vi "Function_Sort Data Array #.vi"(1 "Data Array In":cluster{"Name":string, "Variant Out":variant}[](array[cluster])) -> (0 "Data Array Out":T1)   [LabVIEW 2013]
uses:
  Control/Control_Data Array.ctl
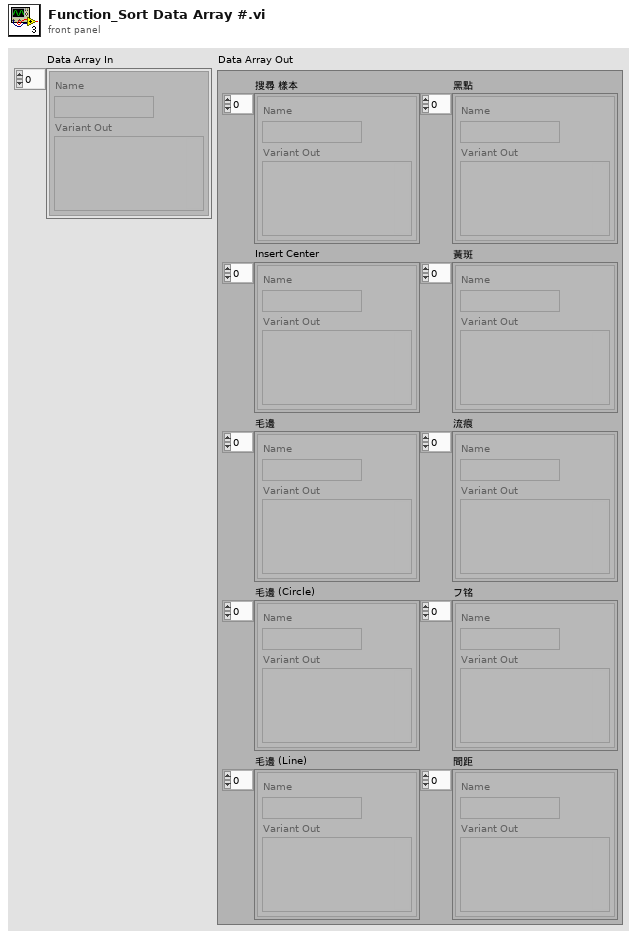
[diagram p1: front panel]
types:
  T1 = typedef "Control_Data Array.ctl" = cluster{"搜尋 樣本":cluster{"Name":string, "Variant Out":variant}[], "Insert Center":cluster{"Name":string, "Variant Out":variant}[], "毛邊":cluster{"Name":string, "Variant Out":variant}[], "毛邊 (Circle)":cluster{"Name":string, "Variant Out":variant}[], "毛邊 (Line)":cluster{"Name":string, "Variant Out":variant}[], "黑點":cluster{"Name":string, "Variant Out":variant}[], "黃斑":cluster{"Name":string, "Variant Out":variant}[], "流痕":cluster{"Name":string, "Variant Out":variant}[], "フ铭":cluster{"Name":string, "Variant Out":variant}[], "間距":cluster{"Name":string, "Variant Out":variant}[]}
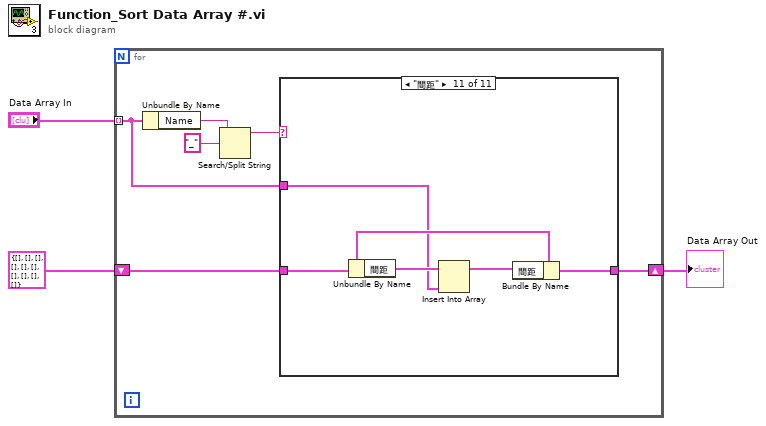
[diagram p0: block diagram]
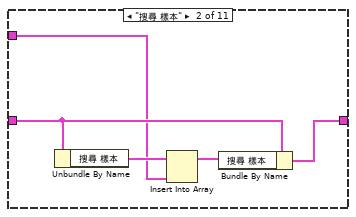
[diagram p3: hidden frame]
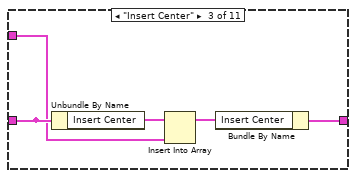
[diagram p4: hidden frame]
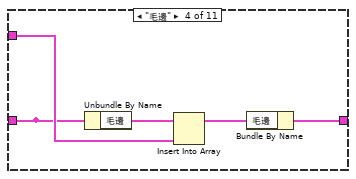
[diagram p5: hidden frame]
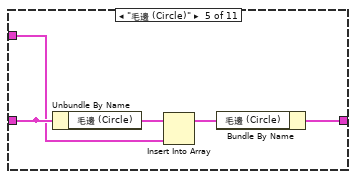
[diagram p6: hidden frame]
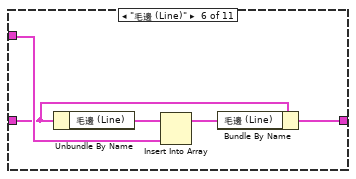
[diagram p7: hidden frame]
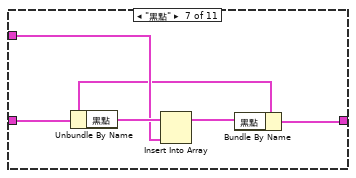
[diagram p8: hidden frame]
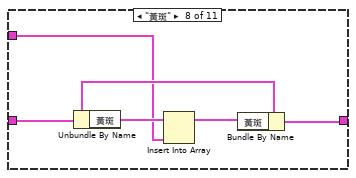
[diagram p9: hidden frame]
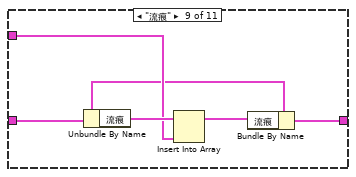
[diagram p10: hidden frame]
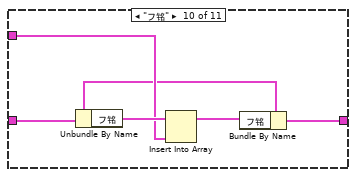
[diagram p11: hidden frame]
diagram:
  n1 = for {
    tunnel: "Data Array In" -> [w7] mode=indexing
    shift-right: [w5] -> w1
    shift-left: T1 {"搜尋 樣本"=[], "Insert Center"=[], "毛邊"=[], "毛邊 (Circle)"=[], "毛邊 (Line)"=[], "黑點"=[], "黃斑"=[], "流痕"=[], "フ铭"=[], "間距"=[]} ("Data Array Out") -> [w6]
    n2 = Unbundle By Name(w7) -> ("Name"=w8:string)
    n3 = Search/Split String(string=w8, search string/char (-)="_") -> (substring before match=w4:string)  [unwired: 1 in, 2 out]
    n4 = case shown="\"間距\"" w4 {
      tunnel: w7 -> [_ w11 w16 w22 w26 w32 w37 w41 w48 w53 w56]
      tunnel: w6 -> [w10 w15 w18 w21 w28 w31 w36 w43 w46 w51 w57]
      tunnel: [w10 w14 w17 w23 w27 w33 w38 w42 w47 w52 w58] -> w5
      frame " - - 選擇檢測項目- - ", Default {
      }
      frame "搜尋 樣本" {
        n5 = Unbundle By Name(w15) -> ("搜尋 樣本"=w13:cluster{"Name":string, "Variant Out":variant}[])
        n6 = Insert Into Array(array=w13, new element=w11) -> (w12:cluster{"Name":string, "Variant Out":variant}[])  [unwired: 1 in]
        n7 = Bundle By Name(cluster=w15, "搜尋 樣本"=w12) -> (w14:T1)
      }
      frame "Insert Center" {
        n8 = Unbundle By Name(w18) -> ("Insert Center"=w20:cluster{"Name":string, "Variant Out":variant}[])
        n9 = Insert Into Array(array=w20, new element=w16) -> (w19:cluster{"Name":string, "Variant Out":variant}[])  [unwired: 1 in]
        n10 = Bundle By Name(cluster=w18, "Insert Center"=w19) -> (w17:T1)
      }
      frame "毛邊" {
        n11 = Unbundle By Name(w21) -> ("毛邊"=w25:cluster{"Name":string, "Variant Out":variant}[])
        n12 = Insert Into Array(array=w25, new element=w22) -> (w24:cluster{"Name":string, "Variant Out":variant}[])  [unwired: 1 in]
        n13 = Bundle By Name(cluster=w21, "毛邊"=w24) -> (w23:T1)
      }
      frame "毛邊 (Circle)" {
        n14 = Unbundle By Name(w28) -> ("毛邊 (Circle)"=w30:cluster{"Name":string, "Variant Out":variant}[])
        n15 = Insert Into Array(array=w30, new element=w26) -> (w29:cluster{"Name":string, "Variant Out":variant}[])  [unwired: 1 in]
        n16 = Bundle By Name(cluster=w28, "毛邊 (Circle)"=w29) -> (w27:T1)
      }
      frame "毛邊 (Line)" {
        n17 = Unbundle By Name(w31) -> ("毛邊 (Line)"=w35:cluster{"Name":string, "Variant Out":variant}[])
        n18 = Insert Into Array(array=w35, new element=w32) -> (w34:cluster{"Name":string, "Variant Out":variant}[])  [unwired: 1 in]
        n19 = Bundle By Name(cluster=w31, "毛邊 (Line)"=w34) -> (w33:T1)
      }
      frame "黑點" {
        n20 = Unbundle By Name(w36) -> ("黑點"=w40:cluster{"Name":string, "Variant Out":variant}[])
        n21 = Insert Into Array(array=w40, new element=w37) -> (w39:cluster{"Name":string, "Variant Out":variant}[])  [unwired: 1 in]
        n22 = Bundle By Name(cluster=w36, "黑點"=w39) -> (w38:T1)
      }
      frame "黃斑" {
        n23 = Unbundle By Name(w43) -> ("黃斑"=w45:cluster{"Name":string, "Variant Out":variant}[])
        n24 = Insert Into Array(array=w45, new element=w41) -> (w44:cluster{"Name":string, "Variant Out":variant}[])  [unwired: 1 in]
        n25 = Bundle By Name(cluster=w43, "黃斑"=w44) -> (w42:T1)
      }
      frame "流痕" {
        n26 = Unbundle By Name(w46) -> ("流痕"=w50:cluster{"Name":string, "Variant Out":variant}[])
        n27 = Insert Into Array(array=w50, new element=w48) -> (w49:cluster{"Name":string, "Variant Out":variant}[])  [unwired: 1 in]
        n28 = Bundle By Name(cluster=w46, "流痕"=w49) -> (w47:T1)
      }
      frame "フ铭" {
        n29 = Unbundle By Name(w51) -> ("フ铭"=w55:cluster{"Name":string, "Variant Out":variant}[])
        n30 = Insert Into Array(array=w55, new element=w53) -> (w54:cluster{"Name":string, "Variant Out":variant}[])  [unwired: 1 in]
        n31 = Bundle By Name(cluster=w51, "フ铭"=w54) -> (w52:T1)
      }
      frame "間距" {
        n32 = Unbundle By Name(w57) -> ("間距"=w60:cluster{"Name":string, "Variant Out":variant}[])
        n33 = Insert Into Array(array=w60, new element=w56) -> (w59:cluster{"Name":string, "Variant Out":variant}[])  [unwired: 1 in]
        n34 = Bundle By Name(cluster=w57, "間距"=w59) -> (w58:T1)
      }
    }
  }
  "Data Array Out" <- w1
